vi "Build Acoustic Task.vi"(8 "error in":errorcluster, 10 "CellInfo":T1[](array[typedef]), 11 "PAS in":refnum<class "PAS.lvclass">) -> (0 "error out":errorcluster, 3 "PAS out":refnum<class "PAS.lvclass">)   [LabVIEW 2014, in "PAS.lvclass"]
doc: "Build the PAS task for measurerments associated with the acoustic analog inputs. The operational values for each of the cell objects contained in the PAS object will be populated first and the measurements will be ordered such that they are in descending cell order and grouped as either microphone or laser diode. The order looks like:\n\n* Cell 1, Mic\n* Cell 2, Mic\n* ....\n* Cell N, Mic\n* Cell 1, Laser\n....\n\nThe name of the task that is created is <B>Acoustic</B> and the task is set to sample coherently and continuously at the config file defined rate. In the original instrument, the PAS uses two S-series cards for 10 measurements (microphone and laser diode)."
uses:
  PAS.lvclass
  Controls/Acoustic IO Record.ctl
  Controls/LasLam.ctl
  Controls/Cell Num.ctl
  Controls/AISigType.ctl
  Controls/Cell Condition.ctl
  PAS.lvclass/PAS.ctl
  Read Cells.vi
  Cell/Write extParams.vi
  Cell/Write l (nm).vi
  Cell/Write Condition.vi
  Cell/PAS Cell.lvclass
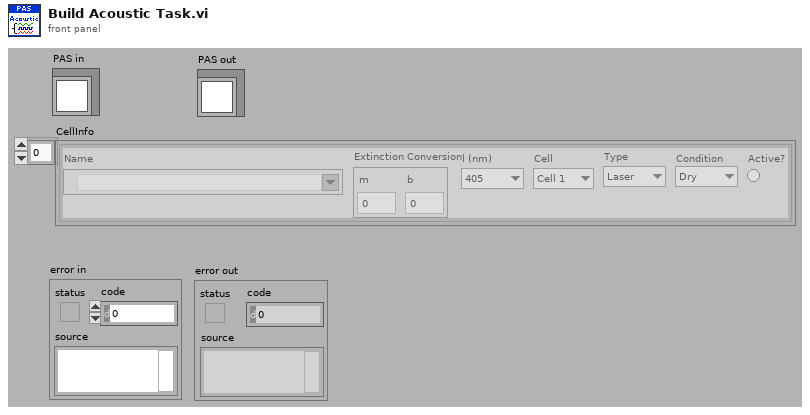
[diagram p1: front panel]
types:
  T1 = typedef "Acoustic IO Record.ctl" = cluster{"Name":tag, "extConv":cluster{"m":dbl, "b":dbl}, "lambda":T2, "Cell":T3, "Type":T4, "Condition":T5, "Active?":bool}
  T2 = typedef "LasLam.ctl" = enum16{"405", "532", "661"}
  T3 = typedef "Cell Num.ctl" = enum16{"Cell 1", "Cell 2", "Cell 3", "Cell 4", "Cell 5", "None"}
  T4 = typedef "AISigType.ctl" = enum16{"Laser", "Microphone"}
  T5 = typedef "Cell Condition.ctl" = enum16{"Dry", "Humidified", "Denuded"}
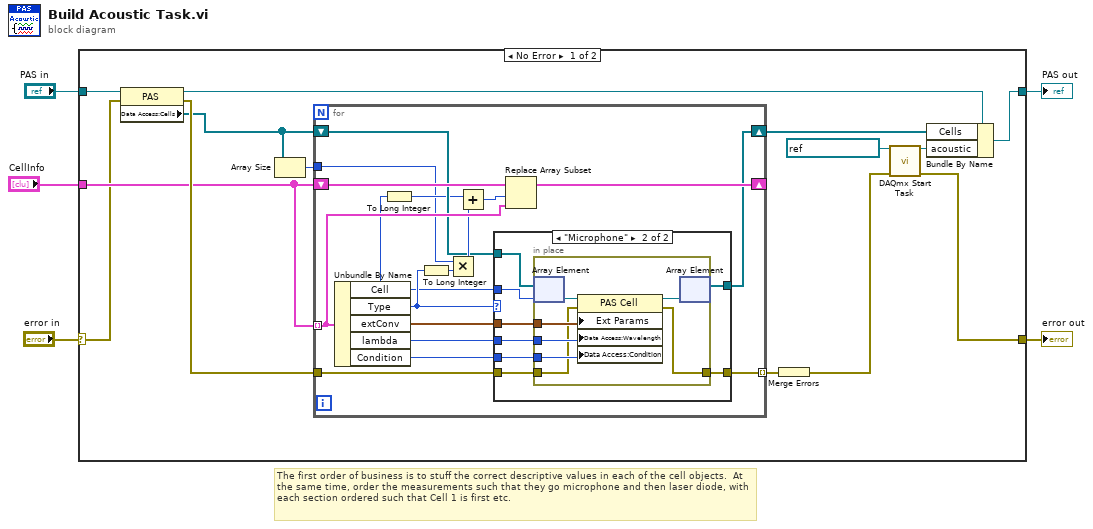
[diagram p0: block diagram]
diagram:
  # "The first order of business is to stuff the correct descriptive values in each of the cell objects.  At the same time, order the measurements such that they go microphone and then laser diode, with each section ordered such that Cell 1 is first etc."
  n1 = case shown="No Error" "error in" {
    selector: "error in" -> [w6 w55]
    tunnel: [w8 w55] -> w4
    tunnel: [w18 w54] -> w2
    tunnel: "PAS in" -> [w16 w54]
    tunnel: "CellInfo" -> [w7 _]
    frame No Error {
      n2 = property class="PAS"(reference=w16, error in=w6) -> (reference out=w15:refnum<class "PAS.lvclass">, error out=w14:errorcluster, "Data Access:Cells"=w13:refnum<class "PAS Cell.lvclass">[])
      n3 = Array Size(array=w13) -> (size(s)=w17:i32)
      n4 = for {
        tunnel: w7 -> [w35] mode=indexing
        shift-right: [w33] -> _
        shift-left: w7 -> [w36]
        shift-right: [w29] -> w19
        shift-left: w13 -> [w30]
        tunnel: w14 -> [w28]
        tunnel: [w27] -> w12 mode=indexing
        tunnel: w17 -> [w21]
        n5 = Unbundle By Name(w35) -> ("Cell"=w20:T3, "Type"=w23:T4, "extConv"=w31:cluster{"m":dbl, "b":dbl}, "lambda"=w25:T2, "Condition"=w26:T5)
        n6 = To Long Integer(number=w20) -> (32bit integer=w24:i32)
        n7 = To Long Integer(number=w23) -> (32bit integer=w22:i32)
        n8 = Multiply(x=w21, y=w22) -> (x*y=w32:i32)
        n9 = Add(x=w24, y=w32) -> (x+y=w34:i32)
        n10 = case shown="\"Microphone\"" w23 {
          tunnel: w20 -> [_ w44]
          tunnel: w31 -> [_ w46]
          tunnel: w30 -> [w38 w45]
          tunnel: [w38 w43] -> w29
          tunnel: w28 -> [w37 w42]
          tunnel: [w37 w39] -> w27
          tunnel: w26 -> [_ w41]
          tunnel: w25 -> [_ w40]
          frame "Laser", Default {
          }
          frame "Microphone" {
            n11 = in-place {
              in-place-border: w46 -> [w50]
              in-place-border: w42 -> [w47]
              in-place-border: w41 -> [w48]
              in-place-border: w40 -> [w49]
              in-place-border: [w51] -> w39
              n12 = in-place-array #1(w45, w44) -> (w53:refnum<class "PAS Cell.lvclass">)
              n13 = property class="PAS Cell"(reference=w53, error in=w47, "Ext Params"=w50, "Data Access:Wavelength"=w49, "Data Access:Condition"=w48) -> (reference out=w52:refnum<class "PAS Cell.lvclass">, error out=w51:errorcluster)
              n14 = in-place-array #1(w52) -> (w43:refnum<class "PAS Cell.lvclass">[])  [unwired: 1 out]
            }
          }
        }
        n15 = Replace Array Subset(array=w36, new element=w35, index=w34) -> (w33:T1[])
      }
      n16 = Merge Errors(w12) -> (w9:errorcluster)
      n17 = call <vilib>:"DAQmx Start Task.vi"("task/channels in"=refnum<k21> "PAS Laser AI" ("DAQmxTasks.acoustic"), "error in"=w9) -> ("task out"=w10:refnum<k21>, "error out"=w8:errorcluster)  [unwired: 12 in]
      n18 = Bundle By Name(cluster=w15, "Cells"=w19, "acoustic"=w10) -> (w18:refnum<class "PAS.lvclass">)
    }
    frame Error {
    }
  }
  "error out" <- w4
  "PAS out" <- w2
